vi "Agilent PWM Read Trigger Source.vi"(7 "Agilent PWM":T1, 8 "error in (no error)":errorcluster, 11 "VISA Resource Name":refnum<visa-resource-name>) -> (0 "error out":errorcluster, 2 "Trigger Source":T2, 3 "dup VISA Resource Name":refnum<visa-resource-name>)   [LabVIEW 2011]
doc: "This VI for the HP 8753 is used to read the sweep type.\n\n0 LINEAR FREQ\n1 LOG FREQ\n2 LIST FREQ\n3 CW TIME\n4 POWER SWEEP"
uses:
  TypeDefs/Agilent PWM Trigger Source.ctl
  TypeDefs/Agilent PWM Instrument Info.ctl
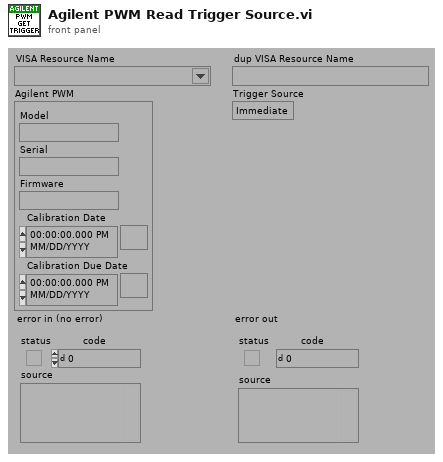
[diagram p1: front panel]
types:
  T1 = typedef "Agilent PWM Instrument Info.ctl" = cluster{"Model":string, "Serial":string, "Firmware":string, "Calibration Date":timestamp, "Calibration Due Date":timestamp}
  T2 = typedef "Agilent PWM Trigger Source.ctl" = enum16{"Immediate", "Bus", "Hold", "Internal", "External"}
  T3 = typedef "Agilent PWM Model.ctl" = enum16{"Not Supported", "E4418X", "E4419X", "U2000X"}
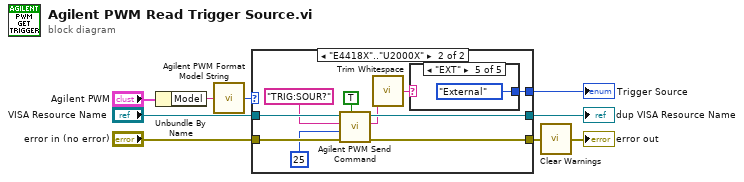
[diagram p0: block diagram]
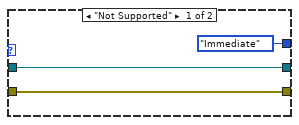
[diagram p2: hidden frame]
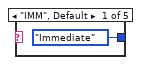
[diagram p3: hidden frame]
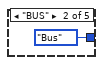
[diagram p4: hidden frame]
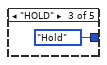
[diagram p5: hidden frame]
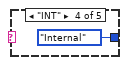
[diagram p6: hidden frame]
diagram:
  n1 = Unbundle By Name("Agilent PWM") -> ("Model"=w4:string)
  n2 = call "Agilent PWM Format Model String.vi"("Model"=w4) -> ("Model"=w2:T3)
  n3 = case shown="\"E4418X\"..\"U2000X\"" w2 {
    tunnel: "error in (no error)" -> [w11 w22]
    tunnel: "VISA Resource Name" -> [w12 w21]
    tunnel: [w12 w18] -> w6
    tunnel: [w11 w17] -> w5
    tunnel: [Agilent_PWM_Trigger_Source."Immediate" ("Trigger Source") w13] -> w1
    frame "Not Supported" {
    }
    frame "E4418X".."U2000X" {
      n4 = call "Agilent PWM Send Command.vi"("Read? (F)"=TRUE, "error in (no error)"=w22, "Byte Count"=u32 25 ("byte count"), "Command"="TRIG:SOUR?" ("write buffer"), "VISA Resource Name"=w21) -> ("error out"=w17:errorcluster, "Data Read"=w16:string, "dup VISA Resource Name"=w18:refnum<visa-resource-name>)  [unwired: 4 out]
      n5 = call <vilib>:"Trim Whitespace.vi"("string"=w16) -> ("trimmed string"=w19:string)  [unwired: 1 in]
      n6 = case shown="\"EXT\"" w19 {
        tunnel: [Agilent_PWM_Trigger_Source."Immediate" ("Trigger Source") Agilent_PWM_Trigger_Source."Bus" ("Trigger Source") Agilent_PWM_Trigger_Source."Hold" ("Trigger Source") Agilent_PWM_Trigger_Source."Internal" ("Trigger Source") Agilent_PWM_Trigger_Source."External" ("Trigger Source")] -> w13
        frame "IMM", Default {
        }
        frame "BUS" {
        }
        frame "HOLD" {
        }
        frame "INT" {
        }
        frame "EXT" {
        }
      }
    }
  }
  "dup VISA Resource Name" <- w6
  "Trigger Source" <- w1
  n7 = call "Clear Warnings.vi"("error in (no error)"=w5) -> ("error out"=→"error out":errorcluster)
